vi "Make Modal Global.vi"() -> ()   [LabVIEW 2018, in "Utilities 1.lvlib"]
uses:
  Utilities 1.lvlib
panel:
  in  "make modal":bool
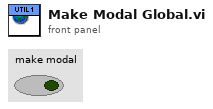
[diagram p1: front panel]
diagram:
